vi "FrameCheck.vi"(8 "Timeout_Indicator":dbl, 11 "Recieved_string_SingleFrame":string) -> (0 "Recieved_Frame_fails_the_check":bool, 3 "Recieved frame_after_error_checks":T1)   [LabVIEW 2021]
panel:
  out "error out":errorcluster
  out "Data_length_error":bool
  out "FrameCheckFail":bool
  out "CRC check error":bool
  out "ClientID_Not_in_range_error":bool
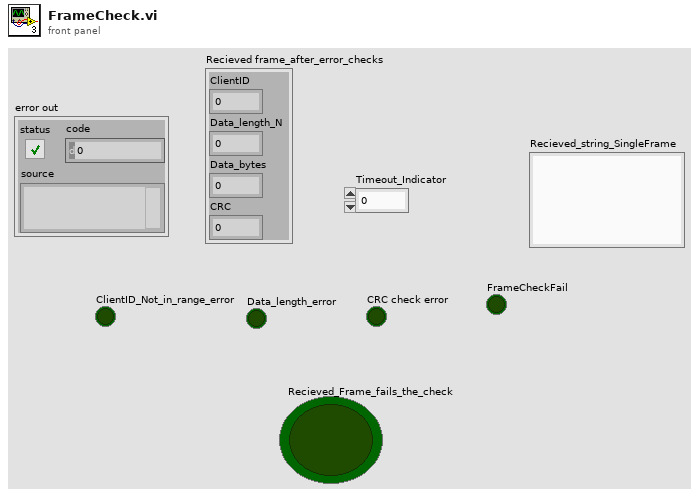
[diagram p1: front panel]
types:
  T1 = cluster{"ClientID":u8, "Data_length_N":i32, "Data_bytes":u8, "CRC":u8}
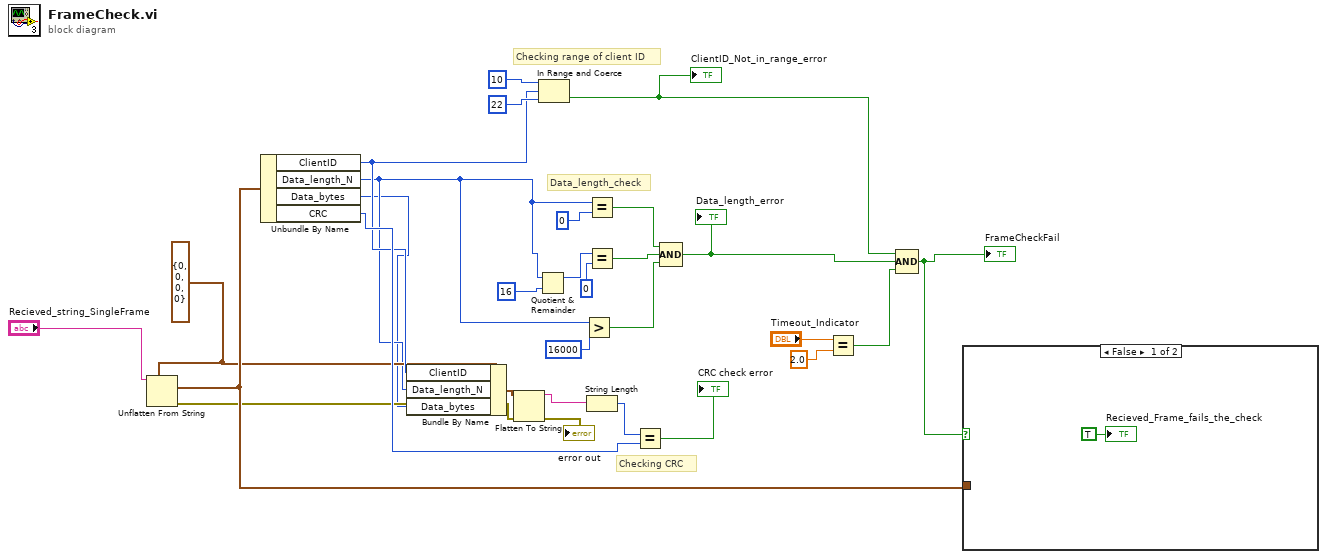
[diagram p0: block diagram]
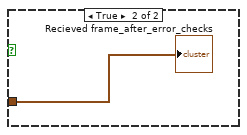
[diagram p2: hidden frame]
diagram:
  w9 = T1 {"ClientID"=0, "Data_length_N"=0, "Data_bytes"=0, "CRC"=0} ("Single_Frame")
  # "Data_length_check"
  # "Checking CRC"
  # "Checking range of client ID"
  n1 = Unflatten From String(type=w9, binary string="Recieved_string_SingleFrame") -> (value=w29:T1, error out=w6:errorcluster)  [unwired: 3 in, 1 out]
  n2 = Unbundle By Name(w29) -> ("ClientID"=w10:u8, "Data_length_N"=w4:i32, "Data_bytes"=w3:u8, "CRC"=w26:u8)
  n3 = Bundle By Name(cluster=w9, "ClientID"=w10, "Data_length_N"=w4, "Data_bytes"=w3) -> (w8:T1)
  n4 = Flatten To String(anything=w8, error in (no error)=w6) -> (data string=w7:string, error out=→"error out":errorcluster)  [unwired: 2 in, 1 out]
  n5 = Quotient & Remainder(x=w4, y=16) -> (x-y*floor(x/y)=w21:i32)  [unwired: 1 out]
  n6 = In Range and Coerce(upper limit=u8 10, x=w10, lower limit=u8 22) -> (In Range?=w1:bool)  [unwired: 1 out]
  "ClientID_Not_in_range_error" <- w1
  n7 = Greater?(x=w4, y=16000) -> (0:w16:bool)
  n8 = Equal?(x=w4, y=0) -> (x = y?=w18:bool)
  n9 = Equal?(x=w21, y=0) -> (x = y?=w17:bool)
  n10 = String Length(string=w7) -> (length=w25:i32)
  n11 = Equal?(x=w25, y=w26) -> (x = y?=→"CRC check error":bool)
  n12 = Compound Arithmetic op=AND(w18, w17, w16) -> (w15:bool)
  "Data_length_error" <- w15
  n13 = Equal?(x="Timeout_Indicator", y=2.0) -> (x = y?=w11:bool)
  n14 = Compound Arithmetic op=AND(w1, w15, w11) -> (w14:bool)
  "FrameCheckFail" <- w14
  n15 = case shown="False" w14 {
    tunnel: w29 -> [_ w31]
    frame False {
      "Recieved_Frame_fails_the_check" <- TRUE ("Recieved_Frame_fails_the_check")
    }
    frame True {
      "Recieved frame_after_error_checks" <- w31
    }
  }
